vi "Front End Resize.vi"(6 "Starting Font":dbl=2570.0 format="%#_13g", 8 "Area to Font Division":dbl=2570.0 format="%#_13g", 9 "Original Text Box Width":i32=60, 10 "NewBnds":T1, 11 "Original Panel Width":u32) -> (2 "New Text Box Width":u64, 3 "New Font Size":dbl)   [LabVIEW 2018, in "Support Library.lvlib"]
uses:
  Support Library.lvlib
  <vilib>/Utility/miscctls.llb/LVRectTypeDef.ctl
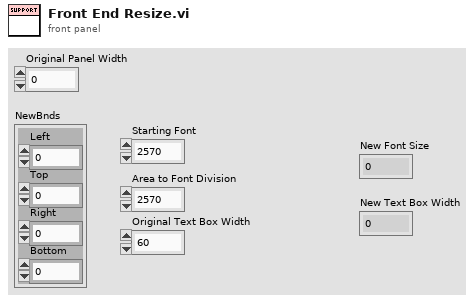
[diagram p1: front panel]
types:
  T1 = typedef "LVRectTypeDef.ctl" = cluster{"Left":i16, "Top":i16, "Right":i16, "Bottom":i16}
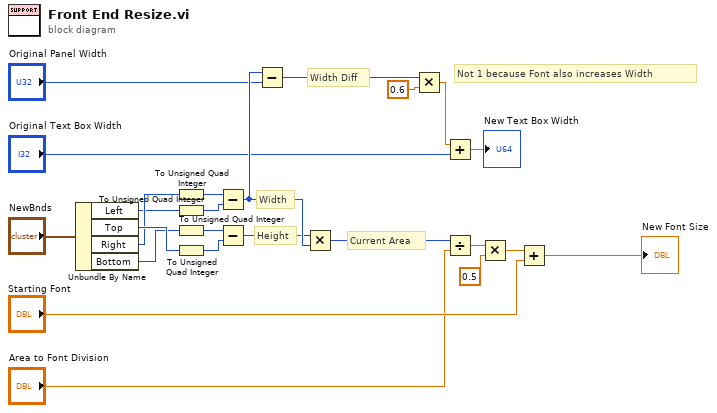
[diagram p0: block diagram]
diagram:
  # "Not 1 because Font also increases Width"
  # "Current Area"
  # "Width Diff"
  # "Height"
  # "Width"
  n1 = Unbundle By Name("NewBnds") -> ("Left"=w13:i16, "Top"=w18:i16, "Right"=w17:i16, "Bottom"=w15:i16)
  n2 = To Unsigned Quad Integer(1:w17) -> (0:w22:u64)
  n3 = To Unsigned Quad Integer(1:w13) -> (0:w14:u64)
  n4 = To Unsigned Quad Integer(1:w15) -> (0:w16:u64)
  n5 = To Unsigned Quad Integer(1:w18) -> (0:w19:u64)
  n6 = Subtract(x=w22, y=w14) -> (x-y=w24:u64)
  n7 = Subtract(x=w16, y=w19) -> (x-y=w23:u64)
  n8 = Subtract(x=w24, y="Original Panel Width") -> (x-y=w3:u64)
  n9 = Multiply(x=w23, y=w24) -> (x*y=w20:u64)
  n10 = Multiply(x=w3, y=0.6) -> (x*y=w10:dbl)
  n11 = Add(x=w10, y="Original Text Box Width") -> (x+y=→"New Text Box Width":dbl)
  n12 = Divide(x=w20, y="Area to Font Division") -> (x/y=w4:dbl)
  n13 = Multiply(x=w4, y=0.5) -> (x*y=w5:dbl)
  n14 = Add(x=w5, y="Starting Font") -> (x+y=→"New Font Size":dbl)
